vi "Initialize.vi"(8 "error in (no error)":errorcluster, 10 "VI Refnum":refnum<vi>, 11 "ControlClassWizard in":refnum<class "QControl Creation Wizard.lvclass">) -> (0 "error out":errorcluster, 3 "ControlClassWizard out":refnum<class "QControl Creation Wizard.lvclass">)   [LabVIEW 2015, in "QControl Creation Wizard.lvclass"]
doc: "<b> </b> <b> </b>\n©2016 Q Software Innovations, LLC (QSI)\nwritten by Quentin Alldredge\nproduced in LabVIEW 2015\n\nsupport@qsoftwareinnovations.com\nwww.qsoftwareinnovations.com\n\nAll rights reserved.\n\nRedistribution and use in source and binary forms, with or without modification, are permitted provided that the following conditions are met:\n\n * Redistributions of source code must retain the above copyright notice, this list of conditions and the following disclaimer.\n * Redistributions in binary form must reproduce the above copyright notice, this list of conditions and the following disclaimer in the documentation and/or other materials provided with the distribution.\n * Neither the name of Q Software Innovations, LLC. nor the names of its contributors may be used to endorse or promote products derived from this software without specific prior written permission.\n\nTHIS SOFTWARE IS PROVIDED BY THE COPYRIGHT HOLDERS AND CONTRIBUTORS \"AS IS\" AND ANY EXPRESS OR IMPLIED WARRANTIES, INCLUDING, BUT NOT LIMITED TO, THE IMPLIED WARRANTIES OF MERCHANTABILITY AND FITNESS FOR A PARTICULAR PURPOSE ARE DISCLAIMED. IN NO EVENT SHALL THE COPYRIGHT OWNER OR CONTRIBUTORS BE LIABLE FOR ANY DIRECT, INDIRECT, INCIDENTAL, SPECIAL, EXEMPLARY, OR CONSEQUENTIAL DAMAGES (INCLUDING, BUT NOT LIMITED TO, PROCUREMENT OF SUBSTITUTE GOODS OR SERVICES; LOSS OF USE, DATA, OR PROFITS; OR BUSINESS INTERRUPTION) HOWEVER CAUSED AND ON ANY THEORY OF LIABILITY, WHETHER IN CONTRACT, STRICT LIABILITY, OR TORT (INCLUDING NEGLIGENCE OR OTHERWISE) ARISING IN ANY WAY OUT OF THE USE OF THIS SOFTWARE, EVEN IF ADVISED OF THE POSSIBILITY OF SUCH DAMAGE."
uses:
  QControl Creation Wizard.lvclass
  QControl Classes/StatusHistory/Direction.ctl
  QControl Creation Wizard.lvclass/QControl Creation Wizard.ctl
  QControl Classes/StatusHistory/Write History Size.vi
  QControl Classes/StatusHistory/Write Direction.vi
  QControl Classes/StatusHistory/Write Least Recent Color.vi
  QControl Classes/StatusHistory/Write Most Recent Color.vi
  QControl Classes/StatusHistory/Write Lock Scrolling.vi
  Dialog/Dialog.lvclass
  QControl Classes/Steps/Steps.lvclass
  QControl Classes/StatusHistory/StatusHistory.lvclass
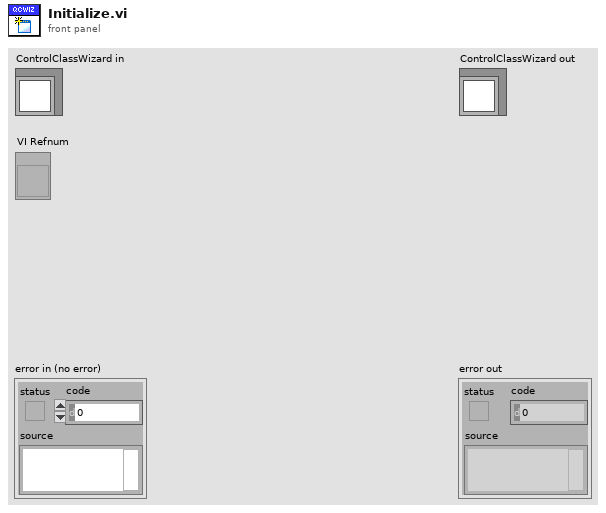
[diagram p1: front panel]
types:
  T1 = typedef "StatusHistory.lvclass/Direction.ctl" = enum16{"Descending", "Ascending"}
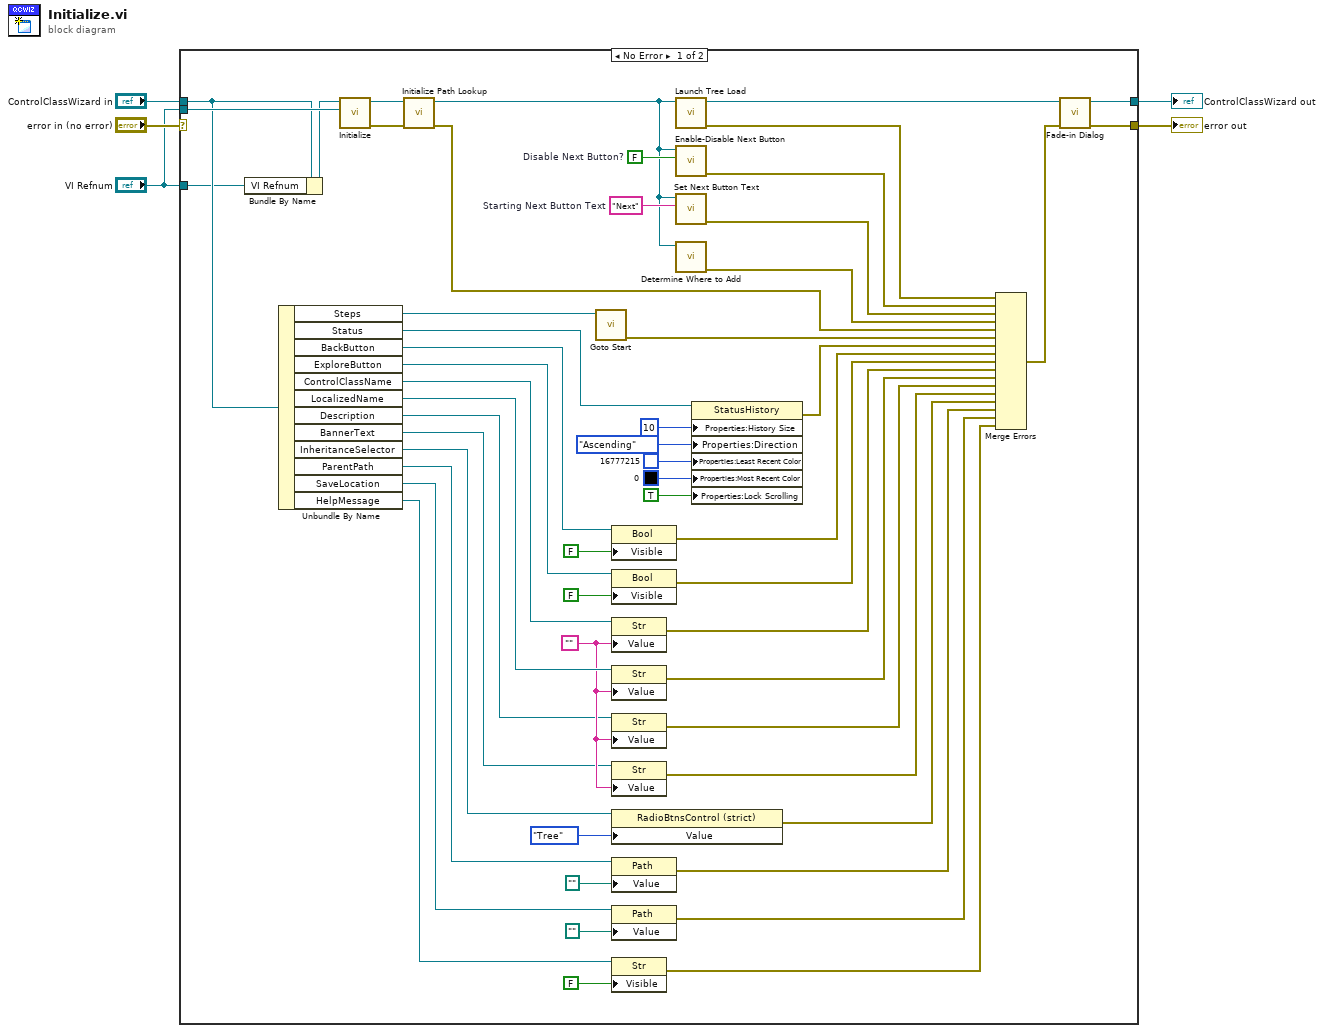
[diagram p0: block diagram]
diagram:
  n1 = case shown="No Error" "error in (no error)" {
    selector: "error in (no error)" -> [_ w61]
    tunnel: [w53 w61] -> w4
    tunnel: [w55 w60] -> w2
    tunnel: "ControlClassWizard in" -> [w36 w60]
    tunnel: "VI Refnum" -> [w37 _]
    tunnel: "VI Refnum" -> [w34 _]
    frame No Error {
      w38 = FALSE  # Disable Next Button?
      w39 = "Next"  # Starting Next Button Text
      w50 = ""
      n2 = Bundle By Name(cluster=w36, "VI Refnum"=w34) -> (w35:refnum<class "QControl Creation Wizard.lvclass">)
      n3 = Unbundle By Name(w36) -> ("Steps"=w59:refnum<class "Steps.lvclass">, "Status"=w28:refnum<class "StatusHistory.lvclass">, "BackButton"=w58:refnum<vi>, "ExploreButton"=w40:refnum<vi>, "ControlClassName"=w52:refnum<vi>, "LocalizedName"=w51:refnum<vi>, "Description"=w49:refnum<vi>, "BannerText"=w48:refnum<vi>, "InheritanceSelector"=w47:refnum<vi>, "ParentPath"=w45:refnum<vi>, "SaveLocation"=w42:refnum<vi>, "HelpMessage"=w26:refnum<vi>)
      n4 = call-parent "Initialize.vi"("VI Refnum"=w37, "Dialog in"=w35) -> ("error out"=w11:errorcluster, "Dialog out"=w10:refnum<class "QControl Creation Wizard.lvclass">)  [unwired: 8 in]
      n5 = call "Initialize Path Lookup.vi"("error in (no error)"=w11, "QControlWizard in"=w10) -> ("error out"=w12:errorcluster, "QControlWizard out"=w7:refnum<class "QControl Creation Wizard.lvclass">)  [unwired: 8 in]
      n6 = call "Goto Start.vi"("Steps in"=w59) -> ("error out"=w9:errorcluster)  [unwired: 9 in, 1 out]
      n7 = property class="Bool"(reference=w58, "Visible"=FALSE ("Control:Visible")) -> (error out=w56:errorcluster)  [unwired: 1 in, 1 out]
      n8 = property class="Bool"(reference=w40, "Visible"=FALSE ("Control:Visible")) -> (error out=w24:errorcluster)  [unwired: 1 in, 1 out]
      n9 = property class="Str"(reference=w52, "Value"=w50) -> (error out=w23:errorcluster)  [unwired: 1 in, 1 out]
      n10 = property class="Str"(reference=w51, "Value"=w50) -> (error out=w22:errorcluster)  [unwired: 1 in, 1 out]
      n11 = property class="Str"(reference=w49, "Value"=w50) -> (error out=w21:errorcluster)  [unwired: 1 in, 1 out]
      n12 = property class="Str"(reference=w48, "Value"=w50) -> (error out=w20:errorcluster)  [unwired: 1 in, 1 out]
      n13 = property class="RadioBtnsControl (strict)"(reference=w47, "Value"=enum32{"Tree", "Path"}."Tree") -> (error out=w19:errorcluster)  [unwired: 1 in, 1 out]
      n14 = property class="Path"(reference=w45, "Value"=path "") -> (error out=w18:errorcluster)  [unwired: 1 in, 1 out]
      n15 = property class="Path"(reference=w42, "Value"=path "") -> (error out=w17:errorcluster)  [unwired: 1 in, 1 out]
      n16 = property class="Str"(reference=w26, "Visible"=FALSE) -> (error out=w16:errorcluster)  [unwired: 1 in, 1 out]
      n17 = call "Launch Tree Load.vi"("QControlWizard in"=w7) -> ("error out"=w8:errorcluster, "QControlWizard out"=w6:refnum<class "QControl Creation Wizard.lvclass">)  [unwired: 9 in]
      n18 = call "Enable-Disable Next Button.vi"("Disable Next Button?"=w38, "QControlWizard in"=w7) -> ("error out"=w13:errorcluster)  [unwired: 8 in, 1 out]
      n19 = call "Set Next Button Text.vi"("Text"=w39, "QControlWizard in"=w7) -> ("error out"=w14:errorcluster)  [unwired: 8 in, 1 out]
      n20 = call "Determine Where to Add.vi"("QControlWizard in"=w7) -> ("error out"=w15:errorcluster)  [unwired: 9 in, 1 out]
      n21 = property class="StatusHistory"(reference=w28, "Properties:History Size"=u32 10 ("History Size"), "Properties:Direction"=Direction."Ascending" ("Direction"), "Properties:Least Recent Color"=u32 16777215, "Properties:Most Recent Color"=u32 0, "Properties:Lock Scrolling"=TRUE ("Lock Scrolling")) -> (error out=w27:errorcluster)  [unwired: 1 in, 1 out]
      n22 = Merge Errors(w8, w13, w14, w15, w12, w9, w27, w56, w24, w23, w22, w21, w20, w19, w18, w17, w16) -> (w54:errorcluster)
      n23 = call "Fade-in Dialog.vi"("error in (no error)"=w54, "Dialog in"=w6) -> ("error out"=w53:errorcluster, "Dialog out"=w55:refnum<class "QControl Creation Wizard.lvclass">)  [unwired: 8 in]
    }
    frame Error {
    }
  }
  "error out" <- w4
  "ControlClassWizard out" <- w2
